vi "Flatten 2D Double Array.vi"(10 "Input Double Matrix":dbl[][](array[numeric])) -> (2 "Flattened Array":dbl[](array[numeric]))   [LabVIEW 2013]
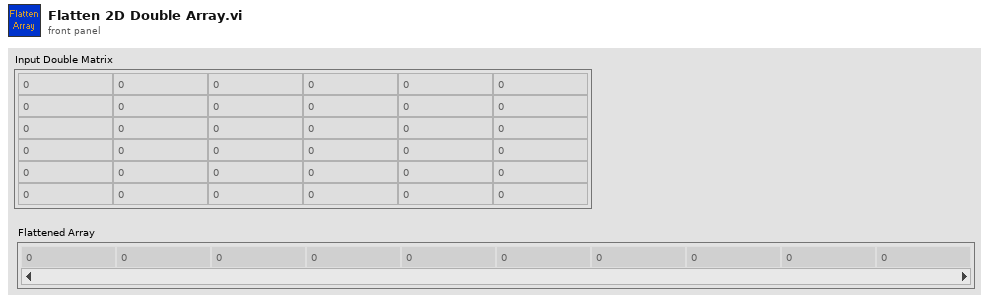
[diagram p1: front panel]
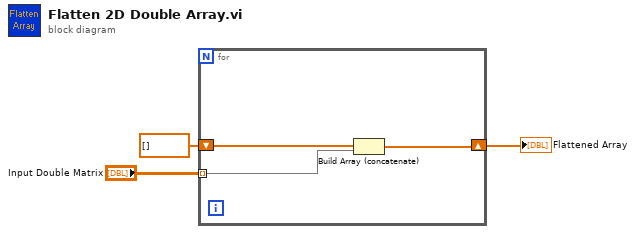
[diagram p0: block diagram]
diagram:
  n1 = for {
    shift-right: [w6] -> w1
    shift-left: dbl[] [] -> [w5]
    tunnel: "Input Double Matrix" -> [w4] mode=indexing
    n2 = Build Array (concatenate)(w5, w4) -> (w6:dbl[])
  }
  "Flattened Array" <- w1
